vi "update-Expgroup.vi"(8 "error in":errorcluster, 10 "String File Paths":string[](array[string]), 11 "EXP group":refnum<class "Experiments_group.lvclass">) -> (0 "error out":errorcluster, 3 "EXP group out":refnum<class "Experiments_group.lvclass">)   [LabVIEW 2020]
uses:
  Classes/Experiments/Experiments_group.lvclass
  Classes/Experiments/Experiment.lvclass
  Classes/Experiments/Experiment.lvclass/Experiment.ctl
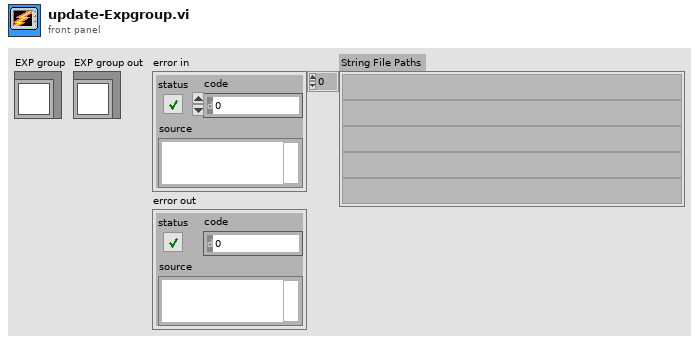
[diagram p1: front panel]
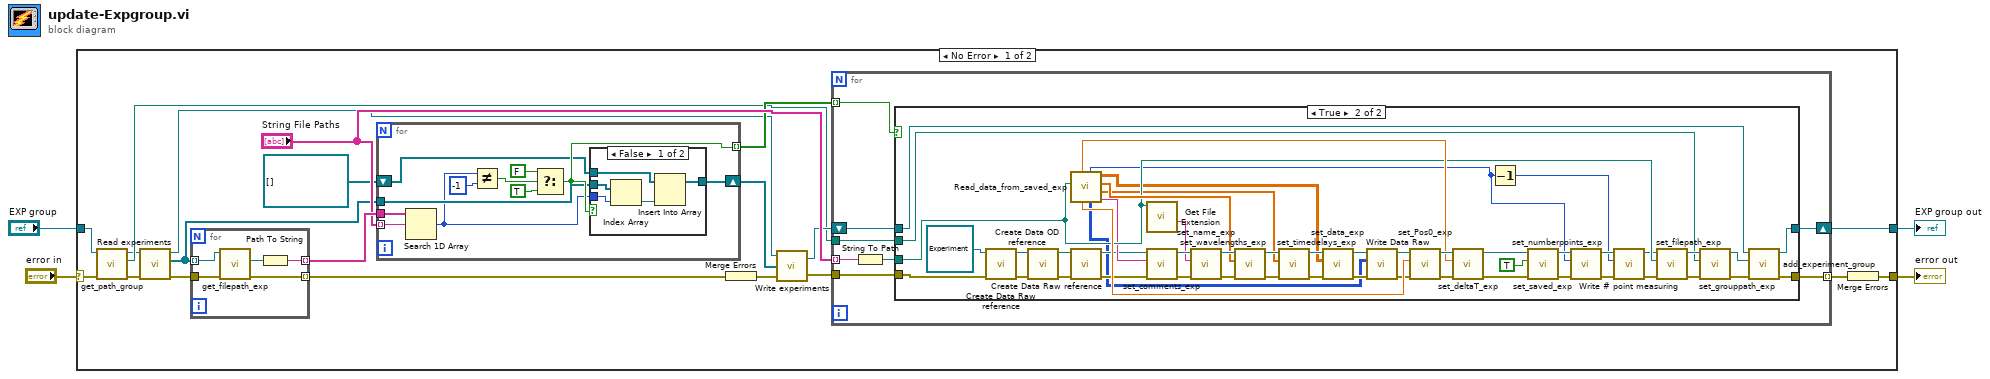
[diagram p0: block diagram]
diagram:
  n1 = case shown="No Error" "error in" {
    selector: "error in" -> [w11 w107]
    tunnel: [w21 w108] -> w4
    tunnel: [w9 w107] -> w1
    tunnel: "EXP group" -> [w14 w108]
    frame No Error {
      n2 = call "get_path_group.vi"("error in (no error)"=w11, "Experiments_group.lvclass in"=w14) -> ("error out"=w22:errorcluster, "Path"=w13:path, "Experiments_group.lvclass out"=w6:refnum<class "Experiments_group.lvclass">)  [unwired: 7 in]
      n3 = call "Read experiments.vi"("error in (no error)"=w22, "Experiments_group.lvclass in"=w6) -> ("error out"=w24:errorcluster, "Experiments"=w12:refnum<class "Experiment.lvclass">[], "Experiments_group.lvclass out"=w5:refnum<class "Experiments_group.lvclass">)  [unwired: 6 in]
      n4 = for {
        tunnel: w12 -> [w106] mode=indexing
        tunnel: w24 -> [w105]
        tunnel: [w104] -> w20 mode=indexing
        tunnel: [w103] -> w23 mode=indexing
        n5 = call "get_filepath_exp.vi"("error in (no error)"=w105, "Experiment.lvclass in"=w106) -> ("error out"=w104:errorcluster, "FilePath"=w102:path)  [unwired: 7 in, 1 out]
        n6 = Path To String(path=w102) -> (string=w103:string)
      }
      n7 = for {
        tunnel: "String File Paths" -> [w90] mode=indexing
        tunnel: w23 -> [w91]
        tunnel: [w89] -> w18 mode=indexing
        tunnel: w12 -> [w88]
        shift-right: [w85] -> w16
        shift-left: refnum<class "Experiment.lvclass">[] [] ("Experiments") -> [w86]
        n8 = Search 1D Array(1D array=w91, element=w90) -> (index of element=w87:i32)  [unwired: 1 in]
        n9 = Not Equal?(x=w87, y=-1) -> (x != y?=w94:bool)
        n10 = Select(t=FALSE, s=w94, f=TRUE) -> (s? t:f=w89:bool)
        n11 = case shown="False" w89 {
          tunnel: w88 -> [w100 _]
          tunnel: w87 -> [w99 _]
          tunnel: w86 -> [w97 w101]
          tunnel: [w96 w101] -> w85
          frame False {
            n12 = Index Array(array=w100, index=w99) -> (element=w98:refnum<class "Experiment.lvclass">)
            n13 = Insert Into Array(array=w97, new element=w98) -> (w96:refnum<class "Experiment.lvclass">[])  [unwired: 1 in]
          }
          frame True {
          }
        }
      }
      n14 = Merge Errors(w20) -> (w8:errorcluster)
      n15 = call-dynamic "Write experiments.vi"("error in (no error)"=w8, "Experiments"=w16, "Experiments_group.lvclass in"=w5) -> ("error out"=w7:errorcluster, "Experiments_group.lvclass out"=w15:refnum<class "Experiments_group.lvclass">)
      n16 = for {
        tunnel: w18 -> [w32] mode=indexing
        tunnel: w13 -> [w31]
        shift-right: [w29] -> w21
        shift-left: w15 -> [w30]
        tunnel: [w28] -> w10 mode=indexing
        tunnel: w7 -> [w27]
        tunnel: "String File Paths" -> [w26] mode=indexing
        n17 = String To Path(string=w26) -> (path=w25:path)
        n18 = case shown="True" w32 {
          tunnel: w25 -> [_ w59]
          tunnel: w31 -> [_ w57]
          tunnel: w30 -> [w34 w82]
          tunnel: [w34 w81] -> w29
          tunnel: [w33 w80] -> w28
          tunnel: w27 -> [w33 w46]
          frame False {
          }
          frame True {
            n19 = call "Create Data Raw reference.vi"("error in (no error)"=w46, "Experiment in"=refnum<class "Experiment.lvclass"> refnum ("Experiment.lvclass")) -> ("error out"=w45:errorcluster, "Experiment out"=w44:refnum<class "Experiment.lvclass">)  [unwired: 8 in]
            n20 = call "Create Data OD reference.vi"("error in (no error)"=w45, "Experiment in"=w44) -> ("error out"=w43:errorcluster, "Experiment out"=w42:refnum<class "Experiment.lvclass">)  [unwired: 8 in]
            n21 = call "Read_data_from_saved_exp.vi"("Path of file"=w59) -> ("Comments"=w48:string, "Time Delays"=w58:dbl[], "Wavelengths"=w63:dbl[], "Data"=w56:dbl[][], "data raw"=w35:i32[][][][], "Number of points"=w50:i32, "Step"=w62:dbl, "Zero time delay"=w61:dbl)  [unwired: 2 in, 1 out]
            n22 = call "Create Data Raw reference.vi"("error in (no error)"=w43, "Experiment in"=w42) -> ("error out"=w40:errorcluster, "Experiment out"=w41:refnum<class "Experiment.lvclass">)  [unwired: 8 in]
            n23 = call <vilib>:"Get File Extension.vi"("file"=w59) -> ("filename without extension"=w65:string)  [unwired: 6 in, 4 out]
            n24 = call "set_comments_exp.vi"("error in (no error)"=w40, "Comments"=w48, "Experiment.lvclass in"=w41) -> ("error out"=w79:errorcluster, "Experiment.lvclass out"=w66:refnum<class "Experiment.lvclass">)  [unwired: 7 in]
            n25 = call "set_name_exp.vi"("error in (no error)"=w79, "Exp name"=w65, "Experiment.lvclass in"=w66) -> ("error out"=w78:errorcluster, "Experiment.lvclass out"=w64:refnum<class "Experiment.lvclass">)  [unwired: 7 in]
            n26 = call "set_wavelengths_exp.vi"("error in (no error)"=w78, "wavelengths"=w63, "Experiment.lvclass in"=w64) -> ("error out"=w71:errorcluster, "Experiment.lvclass out"=w77:refnum<class "Experiment.lvclass">)  [unwired: 7 in]
            n27 = call "set_timedelays_exp.vi"("error in (no error)"=w71, "timedelays"=w58, "Experiment.lvclass in"=w77) -> ("error out"=w55:errorcluster, "Experiment.lvclass out"=w76:refnum<class "Experiment.lvclass">)  [unwired: 7 in]
            n28 = call "set_data_exp.vi"("error in (no error)"=w55, "Data"=w56, "Experiment.lvclass in"=w76) -> ("error out"=w39:errorcluster, "Experiment.lvclass out"=w37:refnum<class "Experiment.lvclass">)  [unwired: 7 in]
            n29 = call-dynamic "Write Data Raw.vi"("error in (no error)"=w39, "Data Raw"=w35, "Experiment in"=w37) -> ("error out"=w38:errorcluster, "Experiment out"=w36:refnum<class "Experiment.lvclass">)  [unwired: 7 in]
            n30 = call "set_Pos0_exp.vi"("error in (no error)"=w38, "Pos0,ps"=w62, "Experiment.lvclass in"=w36) -> ("error out"=w70:errorcluster, "Experiment.lvclass out"=w75:refnum<class "Experiment.lvclass">)  [unwired: 6 in]
            n31 = call "set_deltaT_exp.vi"("error in (no error)"=w70, "deltaTlast"=w61, "Experiment.lvclass in"=w75) -> ("error out"=w69:errorcluster, "Experiment.lvclass out"=w74:refnum<class "Experiment.lvclass">)  [unwired: 6 in]
            n32 = Decrement(x=w50) -> (x-1=w49:i32)
            n33 = call "set_saved_exp.vi"("error in (no error)"=w69, "Saved"=TRUE, "Experiment.lvclass in"=w74) -> ("error out"=w68:errorcluster, "Experiment.lvclass out"=w73:refnum<class "Experiment.lvclass">)  [unwired: 7 in]
            n34 = call "set_numberpoints_exp.vi"("error in (no error)"=w68, "numberpoints"=w50, "Experiment.lvclass in"=w73) -> ("error out"=w53:errorcluster, "Experiment.lvclass out"=w52:refnum<class "Experiment.lvclass">)  [unwired: 6 in]
            n35 = call "Write # point measuring.vi"("error in (no error)"=w53, "# point measuring"=w49, "Experiment in"=w52) -> ("error out"=w54:errorcluster, "Experiment out"=w51:refnum<class "Experiment.lvclass">)  [unwired: 7 in]
            n36 = call "set_filepath_exp.vi"("error in (no error)"=w54, "FilePath"=w59, "Experiment.lvclass in"=w51) -> ("error out"=w67:errorcluster, "Experiment.lvclass out"=w72:refnum<class "Experiment.lvclass">)  [unwired: 7 in]
            n37 = call "set_grouppath_exp.vi"("error in (no error)"=w67, "GroupPath"=w57, "Experiment.lvclass in"=w72) -> ("error out"=w84:errorcluster, "Experiment.lvclass out"=w83:refnum<class "Experiment.lvclass">)  [unwired: 7 in]
            n38 = call-dynamic "add_experiment_group.vi"("error in (no error)"=w84, "Experiment.lvclass"=w83, "Experiments_group.lvclass in"=w82) -> ("error out"=w80:errorcluster, "Experiments_group.lvclass out"=w81:refnum<class "Experiments_group.lvclass">)  [unwired: 7 in]
          }
        }
      }
      n39 = Merge Errors(w10) -> (w9:errorcluster)
    }
    frame Error {
    }
  }
  "EXP group out" <- w4
  "error out" <- w1
